vi "FTW-Endpoint-Initialize.vi"(0 "FTW Endpoint Type":refnum<class "FTW-Endpoint.lvclass">, 11 "error in":errorcluster) -> (4 "FTW Endpoint":refnum<class "FTW-Endpoint.lvclass">, 15 "error out":errorcluster)   [LabVIEW 2012, in "FTW-Actor.lvlib" / "FTW-Endpoint.lvclass"]
uses:
  FTW-Endpoint.lvclass
panel:
  # "Inputs"
  # "Outputs"
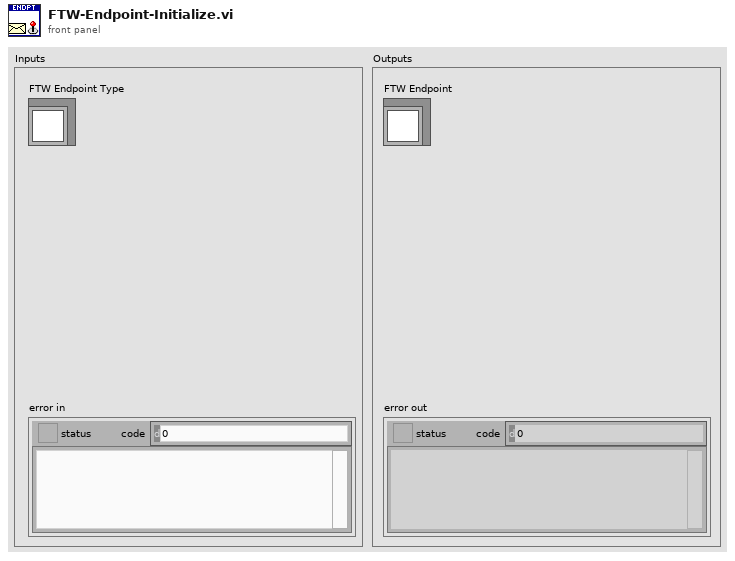
[diagram p1: front panel]
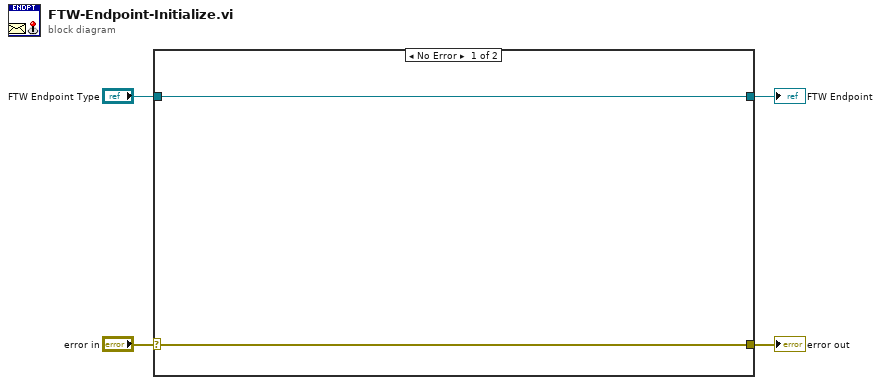
[diagram p0: block diagram]
diagram:
  n1 = case shown="No Error" "error in" {
    selector: "error in" -> [w5 w8]
    tunnel: [w5 w8] -> w4
    tunnel: [w6 w7] -> w2
    tunnel: "FTW Endpoint Type" -> [w6 w7]
    frame No Error {
    }
    frame Error {
    }
  }
  "error out" <- w4
  "FTW Endpoint" <- w2
